vi "Accelerometer Filter.vi"(3 "accelerometer (g)":T1 {"z axis (g)" format="%.3f"; "y axis (g)" format="%.3f"; "x axis (g)" format="%.3f"}) -> (0 "filtered accelerometer (g)":T1 {"z axis (g)" format="%.3f"; "y axis (g)" format="%.3f"; "x axis (g)" format="%.3f"})   [LabVIEW 2018]
uses:
  Accelerometer.ctl
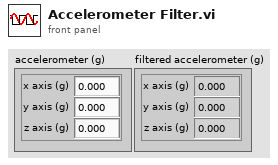
[diagram p1: front panel]
types:
  T1 = typedef "Accelerometer.ctl" = cluster{"x axis (g)":dbl, "y axis (g)":dbl, "z axis (g)":dbl}
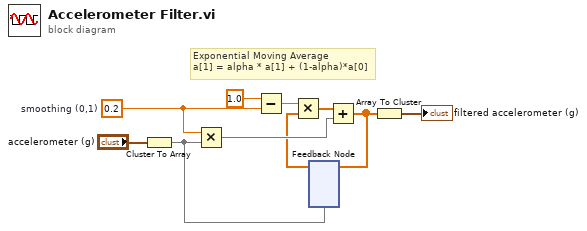
[diagram p0: block diagram]
diagram:
  w1 = 0.2  # smoothing (0,1)
  # "Exponential Moving Average\na[1] = alpha * a[1] + (1-alpha)*a[0]"
  n1 = Cluster To Array(cluster="accelerometer (g)") -> (array=w5:dbl[])
  n2 = Multiply(x=w1, y=w5) -> (x*y=w6:dbl[])
  n3 = Subtract(x=1.0, y=w1) -> (x-y=w8:dbl)
  n4 = feedback #1(w5) -> (w4:dbl[])
  n5 = Multiply(x=w8, y=w4) -> (x*y=w7:dbl[])
  n6 = Add(x=w7, y=w6) -> (x+y=w3:dbl[])
  n7 = feedback-in #1(w3) -> ()
  n8 = Array To Cluster(array=w3) -> (cluster=→"filtered accelerometer (g)":cluster{"[0]":dbl, "[1]":dbl, "[2]":dbl})
